vi "Index Matrices_2011.vi"(3 "Image In":dbl[][](array[numeric])) -> (0 "M(j)":i32[][](array[numeric]), 1 "M(i)":i32[][](array[numeric]))   [LabVIEW 2013]
uses:
  NI_AALBase.lvlib
panel:
  out "Array":dbl[][](array[numeric])
  out "Ramp Pattern":dbl[](array[numeric])
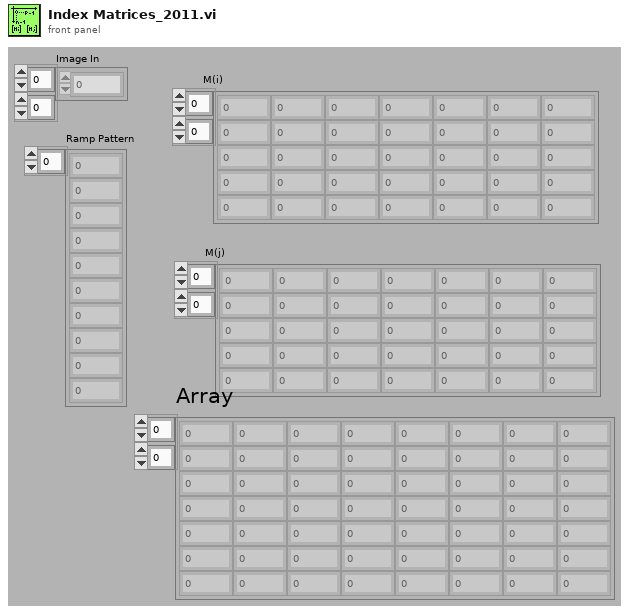
[diagram p1: front panel]
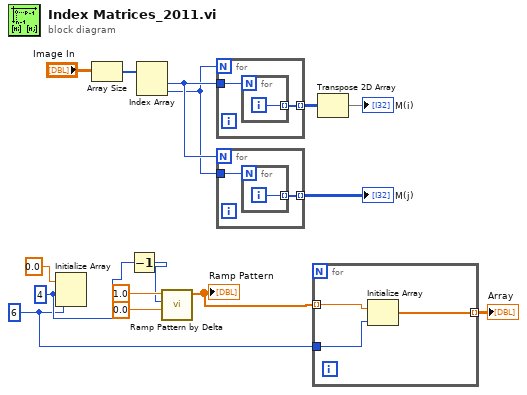
[diagram p0: block diagram]
diagram:
  w3 = 6 ("dimension size")
  w6 = 4 ("dimension size")
  n1 = Initialize Array(0.0 ("element"), w6, w3) -> ()  [unwired: 1 out]
  n2 = Array Size(array="Image In") -> (size(s)=w15:i32[])
  n3 = Decrement(x=w6) -> (x-1=w5:i32)
  n4 = Index Array(array=w15) -> (element #1=w13:i32, element #2=w12:i32)  [unwired: 2 in]
  n5 = call "Ramp Pattern by Delta.vi"("start"=0.0, "end"=w5, "delta"=1.0) -> ("Ramp Pattern"=w4:dbl[])  [unwired: 6 in, 2 out]
  "Ramp Pattern" <- w4
  n6 = for {
    N: w12 -> [_]
    tunnel: w13 -> [w17]
    tunnel: [w16] -> w14 mode=indexing
    n7 = for {
      N: w17 -> [_]
      tunnel: [w18] -> w16 mode=indexing
      i -> [w18]
    }
  }
  n8 = for {
    N: w13 -> [_]
    tunnel: w12 -> [w20]
    tunnel: [w19] -> w10 mode=indexing
    n9 = for {
      N: w20 -> [_]
      tunnel: [w21] -> w19 mode=indexing
      i -> [w21]
    }
  }
  "M(j)" <- w10
  n10 = for {
    tunnel: w4 -> [w24] mode=indexing
    tunnel: w3 -> [w23]
    tunnel: [w22] -> w2 mode=indexing
    n11 = Initialize Array(w24, w23) -> (w22:dbl[])
  }
  "Array" <- w2
  n12 = Transpose 2D Array(2D array=w14) -> (transposed array=→"M(i)":i32[][])
